vi "Guidance.vi"   [LabVIEW 2014, in "Guidance Library.lvlib" / "Guidance.lvclass"]
uses:
  Guidance.lvclass
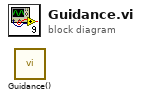
[diagram p0: block diagram]
diagram:
  n1 = call "Guidance().vi"() -> ()  [unwired: 11 in, 1 out]
